vi "MotorWaitIdle.vi"(3 "Motor":string, 9 "error in (no error)":errorcluster) -> (0 "Motor out":string, 6 "error out":errorcluster)   [LabVIEW 2009]
uses:
  Controls/MotorStatus.ctl
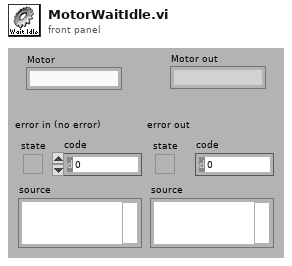
[diagram p1: front panel]
types:
  T1 = typedef "MotorStatus.ctl" = cluster{"Managed?":bool, "Position":i32, "Name":string, "Status":enum16{"OFF", "IDLE", "MOVING", "HOMING"}}
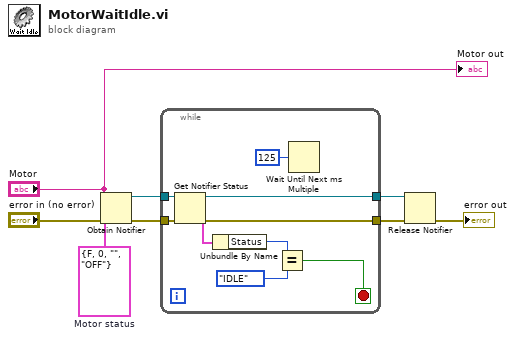
[diagram p0: block diagram]
diagram:
  w1 = T1 {"Managed?"=FALSE, "Position"=0, "Name"="", "Status"=enum."OFF"}  # Motor status
  n1 = Obtain Notifier(name (unnamed)="Motor", notification data type=w1, error in (no error)="error in (no error)") -> (notifier out=w4:refnum<notifier>, error out=w5:errorcluster)  [unwired: 1 in, 1 out]
  n2 = while {
    tunnel: [w17] -> w7
    tunnel: [w16] -> w6
    tunnel: w5 -> [w15]
    tunnel: w4 -> [w14]
    stop <- w10 stop-if-true
    n3 = Get Notifier Status(notifier=w14, error in (no error)=w15) -> (notifier out=w17:refnum<notifier>, current notification=w13:T1, error out=w16:errorcluster)  [unwired: 2 out]
    n4 = Unbundle By Name(w13) -> ("Status"=w12:enum16{"OFF", "IDLE", "MOVING", "HOMING"})
    n5 = Equal?(x=w12, y=enum16{"OFF", "IDLE", "MOVING", "HOMING"}."IDLE" ("Status")) -> (x = y?=w10:bool)
    n6 = Wait Until Next ms Multiple(millisecond multiple=u32 125 ("n millisecondes")) -> ()  [unwired: 1 out]
  }
  n7 = Release Notifier(notifier=w7, error in (no error)=w6) -> (error out=→"error out":errorcluster)  [unwired: 3 out]
  "Motor out" <- "Motor"
